vi "A170316-11_config.vi"() -> ()   [LabVIEW 2020]
uses:
  Global_Variable/Global.vi
  Database/Global1.vi
  <vilib>/Utility/config.llb/NI_LVConfig.lvlib
panel:
  in  "选项卡控件":enum32{"参数", "备用参数", "产品管理"}(tab)
  in  "参数设定":string[][](table)=[["", "", "", ""], ["", "", "", ""]]
  in  "删除":bool
  in  "确定":bool
  in  "添加":bool
  in  "退出":bool
  in  "更新":bool
  in  "产品型号":string(combo)
  in  "请输入添加的产品名称":string
  in  "请选择要删除的产品":string(combo)
  # "激光打标机"
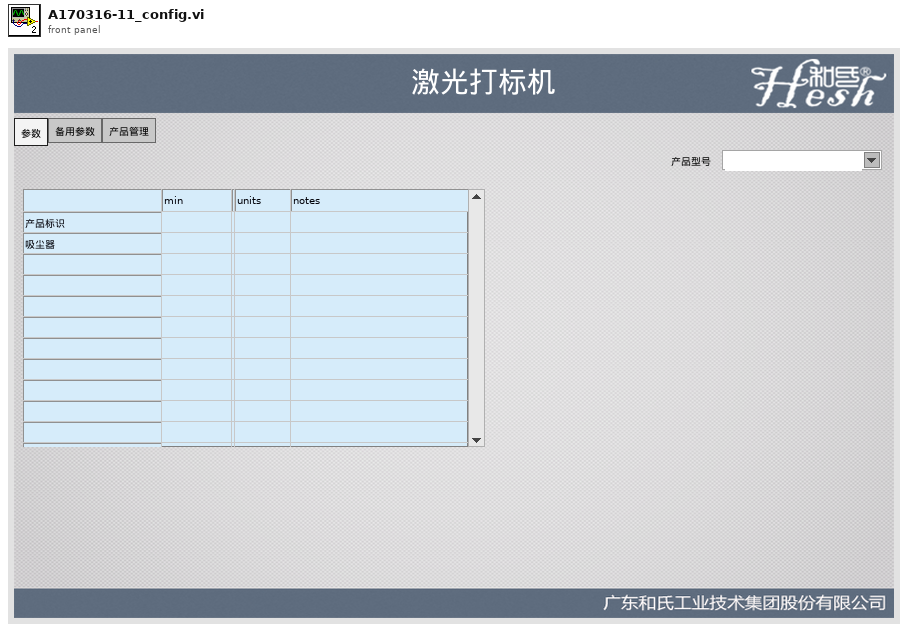
[diagram p1: front panel]
types:
  T1 = typedef "NI_LVConfig.lvlib/Config Data RefNum.ctl" = refnum<k1>
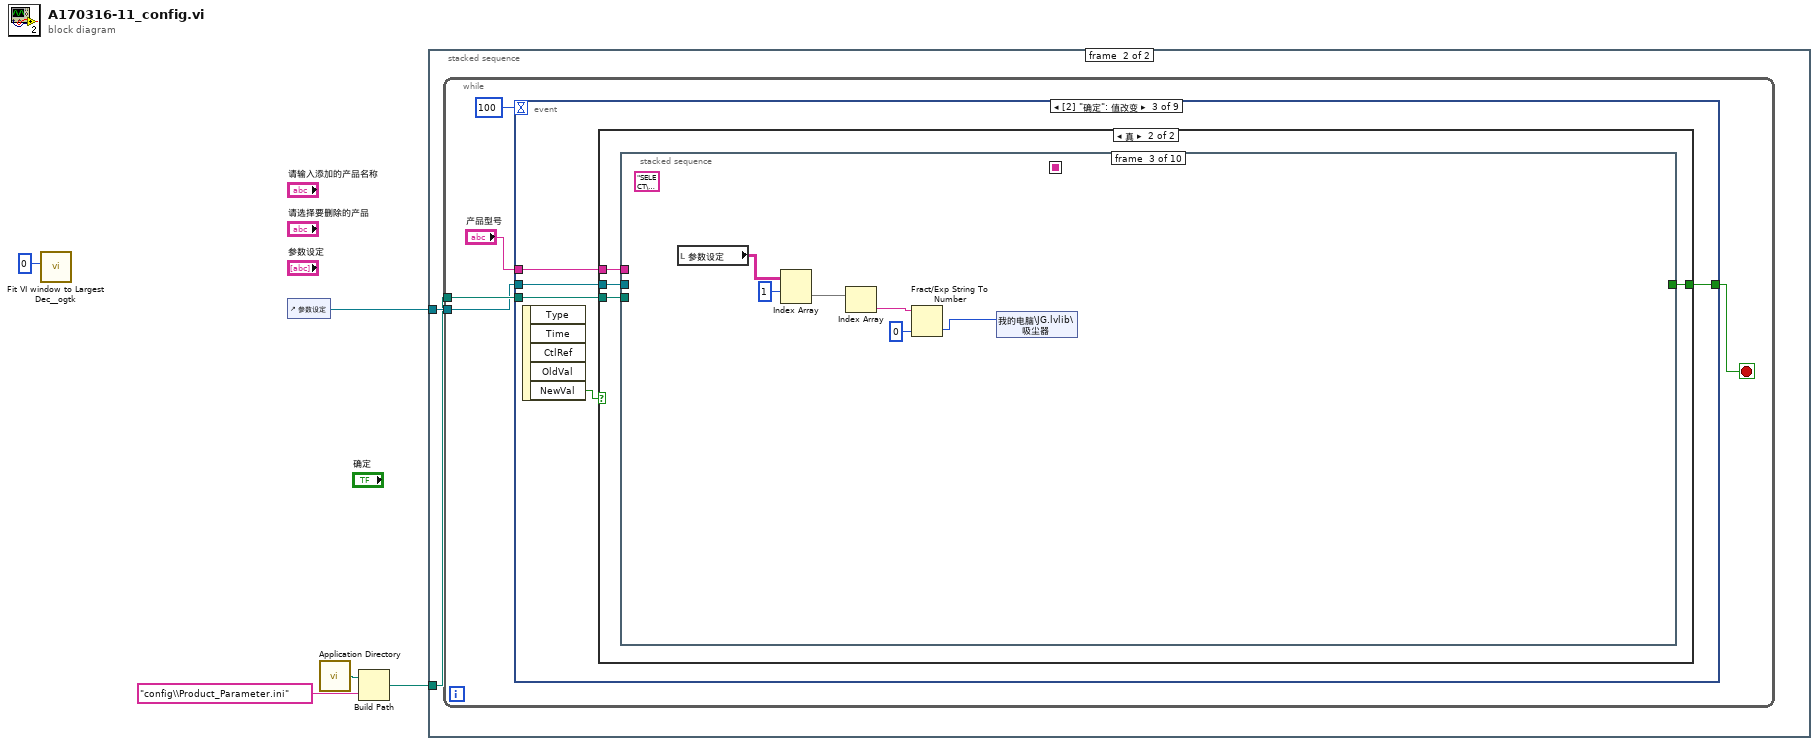
[diagram p0: block diagram]
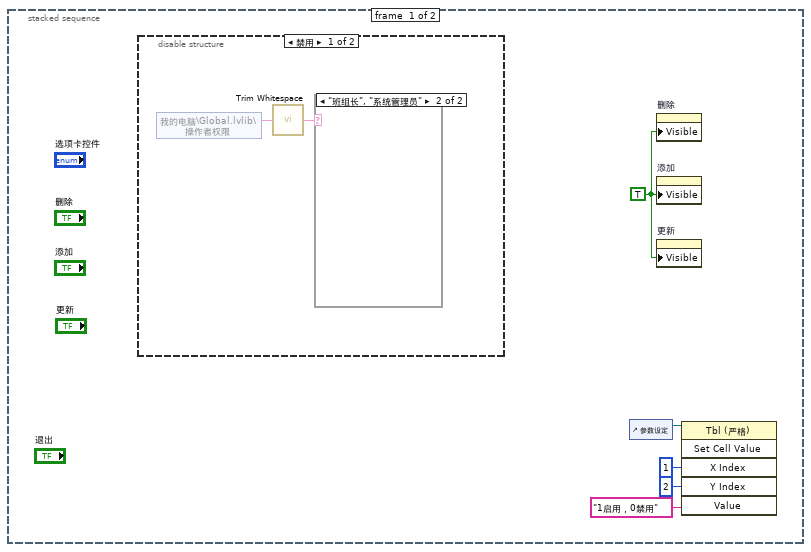
[diagram p2: hidden frame]
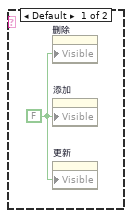
[diagram p3: hidden frame]
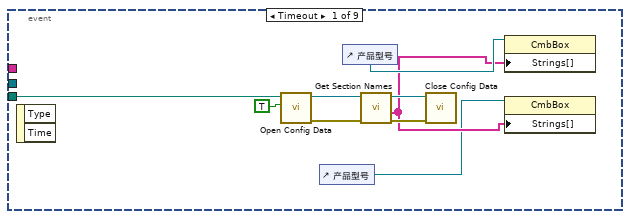
[diagram p5: hidden frame]
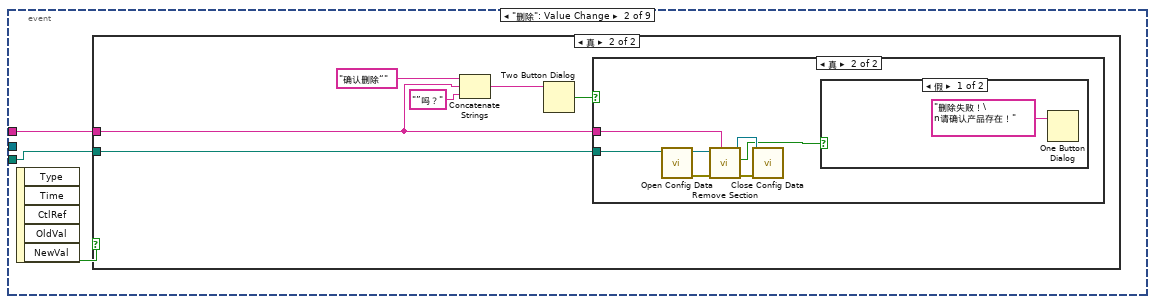
[diagram p6: hidden frame]
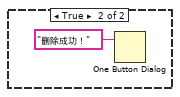
[diagram p9: hidden frame]
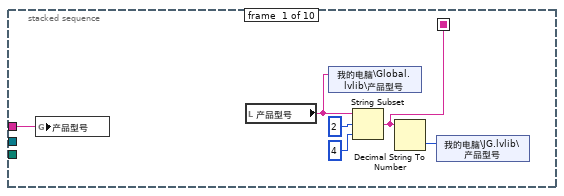
[diagram p11: hidden frame]
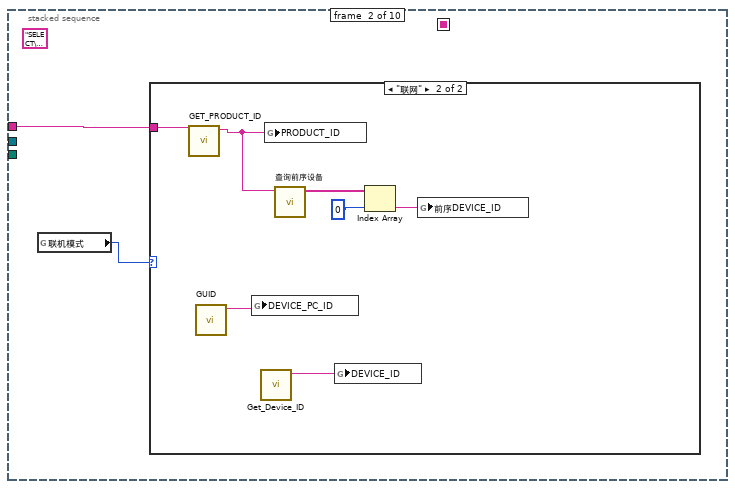
[diagram p12: hidden frame]
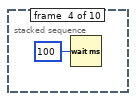
[diagram p14: hidden frame]
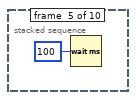
[diagram p15: hidden frame]
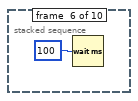
[diagram p16: hidden frame]
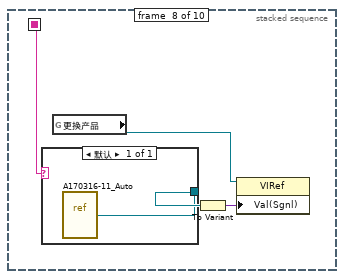
[diagram p18: hidden frame]
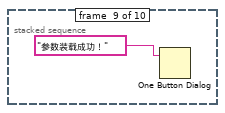
[diagram p19: hidden frame]
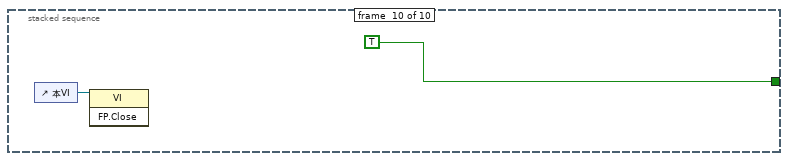
[diagram p20: hidden frame]
diagram:
  n1 = call <userlib>:"Fit VI window to Largest Dec__ogtk.vi"("border spacing (2 px)"=0) -> ()  [unwired: 5 in, 2 out]
  n2 = control-ref of="参数设定"() -> (w1:refnum<vi>)
  n3 = call <vilib>:"Application Directory.vi"() -> ("Application Directory"=w5:path)
  n4 = Build Path(base path=w5, name or relative path="config\\Product_Parameter.ini" ("名称或相对路径")) -> (appended path=w3:path)
  n5 = stacked-sequence {
    tunnel: w1 -> [_ w15]
    tunnel: w3 -> [_ w14]
    frame #0 {
      w10 = TRUE ("可见")
      n6 = disable-structure shown="禁用" {
        frame Disabled {
          n7 = shared-variable "我的电脑\\Global.lvlib\\操作者权限"() -> (w12:string)  [unwired: 1 in, 1 out]
          n8 = call <vilib>:"Trim Whitespace.vi"("string"=w12) -> ("trimmed string"=w11:string)  [unwired: 1 in]
          n9 = case shown="\"班组长\", \"系统管理员\"" w11 {
            frame Default {
              w13 = FALSE ("可见")
              n10 = property on="删除" class="Bool (严格)"("Visible"=w13) -> ()  [unwired: 2 in, 2 out]
              n11 = property on="添加" class="Bool (严格)"("Visible"=w13) -> ()  [unwired: 2 in, 2 out]
              n12 = property on="更新" class="Bool (严格)"("Visible"=w13) -> ()  [unwired: 2 in, 2 out]
            }
            frame "班组长", "系统管理员" {
            }
          }
        }
        frame Enabled {
        }
      }
      n13 = control-ref of="参数设定"() -> (w9:refnum<vi>)
      n14 = property on="删除" class="Bool (严格)"("Visible"=w10) -> ()  [unwired: 2 in, 2 out]
      n15 = property on="添加" class="Bool (严格)"("Visible"=w10) -> ()  [unwired: 2 in, 2 out]
      n16 = property on="更新" class="Bool (严格)"("Visible"=w10) -> ()  [unwired: 2 in, 2 out]
      n17 = invoke class="Tbl (严格)" method="Set Cell Value"(reference=w9, "X Index"=1 ("X索引"), "Y Index"=2 ("Y索引"), "Value"="1启用，0禁用" ("值")) -> ()  [unwired: 2 in, 6 out]
    }
    frame #1 {
      n18 = while {
        tunnel: w14 -> [w20]
        tunnel: w15 -> [w18]
        stop <- w19 stop-if-true
        n19 = event shown="[2] \"确定\": 值改变" {
          selector: _ -> [_ _ _ _ _ _ _ _ _]
          dyn-events: _ -> [_ _ _ _ _ _ _ _ _]
          timeout: 100 -> [_ _ _ _ _ _ _ _ _]
          tunnel: w20 -> [w24 w32 w49 w94 w110 _ w127 _ _]
          tunnel: [_ _ w51 _ _ TRUE _ _ TRUE] -> w19
          tunnel: w18 -> [_ _ w50 w95 w111 _ w126 _ _]
          tunnel: "产品型号" -> [_ w30 w48 w89 _ _ _ _ _]
          event Timeout {
            n20 = event-data() -> ()  [unwired: 1 in, 2 out]
            n21 = call <vilib>:"Open Config Data.vi"("create file if necessary (T)"=TRUE, "configuration file path"=w24) -> ("error out"=w26:errorcluster, "refnum"=w25:T1)  [unwired: 7 in, 1 out]
            n22 = control-ref of="产品型号"() -> (w21:refnum<vi>)
            n23 = control-ref of="产品型号"() -> (w23:refnum<vi>)
            n24 = call <vilib>:"Get Section Names.vi"("error in (no error)"=w26, "refnum"=w25) -> ("error out"=w28:errorcluster, "section names"=w22:string[], "refnum out"=w27:T1)  [unwired: 7 in]
            n25 = call <vilib>:"Close Config Data.vi"("error in (no error)"=w28, "refnum"=w27) -> ()  [unwired: 8 in, 2 out]
            n26 = property on="属性节点" class="CmbBox"(reference=w23, "Strings[]"=w22) -> ()  [unwired: 1 in, 2 out]
            n27 = property on="属性节点" class="CmbBox"(reference=w21, "Strings[]"=w22) -> ()  [unwired: 1 in, 2 out]
          }
          event "删除": Value Change {
            n28 = event-data() -> ("NewVal"=w31:bool)  [unwired: 1 in, 4 out]
            n29 = case shown="真" w31 {
              tunnel: w32 -> [_ w34]
              tunnel: w30 -> [_ w33]
              frame False {
              }
              frame True {
                n30 = Concatenate Strings("确认删除“", w33, "”吗？") -> (w36:string)
                n31 = Two Button Dialog(message=w36) -> (T button?=w35:bool)  [unwired: 2 in]
                n32 = case shown="真" w35 {
                  tunnel: w34 -> [_ w40]
                  tunnel: w33 -> [_ w39]
                  frame False {
                  }
                  frame True {
                    n33 = call <vilib>:"Open Config Data.vi"("configuration file path"=w40) -> ("error out"=w42:errorcluster, "refnum"=w45:T1)  [unwired: 8 in, 1 out]
                    n34 = call <vilib>:"Remove Section.vi"("section"=w39, "error in (no error)"=w42, "refnum"=w45) -> ("error out"=w44:errorcluster, "section exists?"=w41:bool, "refnum out"=w43:T1)  [unwired: 6 in]
                    n35 = call <vilib>:"Close Config Data.vi"("error in (no error)"=w44, "refnum"=w43) -> ()  [unwired: 8 in, 2 out]
                    n36 = case shown="假" w41 {
                      frame False {
                        n37 = One Button Dialog(message="删除失败！\n请确认产品存在！" ("消息")) -> ()  [unwired: 1 in, 1 out]
                      }
                      frame True {
                        n38 = One Button Dialog(message="删除成功！" ("消息")) -> ()  [unwired: 1 in, 1 out]
                      }
                    }
                  }
                }
              }
            }
          }
          event "确定": Value Change {
            n39 = event-data() -> ("NewVal"=w52:bool)  [unwired: 1 in, 4 out]
            n40 = case shown="真" w52 {
              tunnel: [_ w56] -> w51
              tunnel: w50 -> [_ w55]
              tunnel: w49 -> [_ w54]
              tunnel: w48 -> [_ w53]
              frame False {
              }
              frame True {
                n41 = stacked-sequence {
                  seq-local: [w62 _ _ _ _ _ _ _ _ _] -> [_ _ _ _ _ _ _ w84 _ _]
                  tunnel: [_ _ _ _ _ _ _ _ _ TRUE] -> w56
                  tunnel: w55 -> [_ _ _ _ _ _ _ _ _ _]
                  tunnel: w54 -> [_ _ _ _ _ _ _ _ _ _]
                  tunnel: w53 -> [w57 w64 _ _ _ _ _ _ _ _]
                  frame #0 {
                    n42 = global write "Global.vi" "产品型号"(w57) -> ()
                    n43 = local read "产品型号"() -> (w61:string)
                    n44 = shared-variable "我的电脑\\Global.lvlib\\产品型号"(w61) -> ()  [unwired: 1 in, 1 out]
                    n45 = String Subset(string=w61, offset (0)=u16 2 ("偏移量(0)"), length (rest)=u16 4 ("长度（剩余）")) -> (substring=w62:string)
                    n46 = Decimal String To Number(string=w62) -> (number=w58:i32)  [unwired: 2 in, 1 out]
                    n47 = shared-variable "我的电脑\\JG.lvlib\\产品型号"(w58) -> ()  [unwired: 1 in, 1 out]
                  }
                  frame #1 {
                    (unwired) "SELECT\ndbo.[Product].USER_ID\nFROM\ndbo.[Product]\nWHERE\ndbo.[Product].PRODUCT_NAME = '%s'" ("格式字符串")
                    n48 = global read "Global1.vi" "联机模式"() -> (w63:enum16{"单机", "联网"})
                    n49 = case shown="\"联网\"" w63 {
                      tunnel: w64 -> [_ w70]
                      frame "单机", Default {
                      }
                      frame "联网" {
                        n50 = call "GET_PRODUCT_ID.vi"("PRODFUCT_NAME"=w70) -> ("PRODUCT_ID"=w69:string)  [unwired: 10 in]
                        n51 = call "GUID.vi"() -> ("trimmed string"=w71:string)  [unwired: 11 in]
                        n52 = global write "Global1.vi" "DEVICE_PC_ID"(w71) -> ()
                        n53 = call "Get_Device_ID.vi"() -> ("Device_ID"=w65:string)  [unwired: 10 in, 1 out]
                        n54 = global write "Global1.vi" "PRODUCT_ID"(w69) -> ()
                        n55 = call "查询前序设备.vi"("PRODUCT_ID"=w69) -> ("前序工位"=w68:string[])  [unwired: 10 in]
                        n56 = global write "Global1.vi" "DEVICE_ID"(w65) -> ()
                        n57 = Index Array(array=w68, index=0 ("索引")) -> (element=w66:string)
                        n58 = global write "Global1.vi" "前序DEVICE_ID"(w66) -> ()
                      }
                    }
                  }
                  frame #2 {
                    (unwired) "SELECT\ndbo.[Product].USER_ID\nFROM\ndbo.[Product]\nWHERE\ndbo.[Product].PRODUCT_NAME = '%s'" ("格式字符串")
                    n59 = local read "参数设定"() -> (w77:string[][])
                    n60 = Index Array(array=w77, index (row)=1 ("索引 (行)")) -> (element=w76:string[])  [unwired: 1 in]
                    n61 = Index Array(array=w76) -> (element=w74:string)  [unwired: 1 in]
                    n62 = Fract/Exp String To Number(string=w74, default (0 dbl)=0 ("默认(0 DBL)")) -> (number=w73:i32)  [unwired: 2 in, 1 out]
                    n63 = shared-variable "我的电脑\\JG.lvlib\\吸尘器"(w73) -> ()  [unwired: 1 in, 1 out]
                  }
                  frame #3 {
                    n64 = Wait (ms)(milliseconds to wait=u32 100) -> ()  [unwired: 1 out]
                  }
                  frame #4 {
                    n65 = Wait (ms)(milliseconds to wait=u32 100) -> ()  [unwired: 1 out]
                  }
                  frame #5 {
                    n66 = Wait (ms)(milliseconds to wait=u32 100) -> ()  [unwired: 1 out]
                  }
                  frame #6 {
                  }
                  frame #7 {
                    n67 = case shown="默认" w84 {
                      tunnel: [w85] -> w81
                      frame 默认 {
                        n68 = vi-ref "A170316-11_Auto.vi"() -> (w85:refnum<vi>)
                      }
                    }
                    n69 = global read "Global.vi" "更换产品"() -> (w83:refnum<vi>)
                    n70 = To Variant(anything=w81) -> (Variant=w82:variant)
                    n71 = property class="VIRef"(reference=w83, "Val(Sgnl)"=w82) -> ()  [unwired: 1 in, 2 out]
                  }
                  frame #8 {
                    n72 = One Button Dialog(message="参数装载成功！" ("消息")) -> ()  [unwired: 1 in, 1 out]
                  }
                  frame #9 {
                    n73 = control-ref of="本VI"() -> (w87:refnum<vi>)
                    n74 = invoke class="VI" method="FP.Close"(reference=w87) -> ()  [unwired: 2 in, 3 out]
                  }
                }
              }
            }
          }
          event "添加": Value Change {
            n75 = event-data() -> ("NewVal"=w93:bool)  [unwired: 1 in, 4 out]
            n76 = local read "产品型号"() -> (w90:string)
            n77 = call <vilib>:"Trim Whitespace.vi"("string"=w90) -> ("trimmed string"=w91:string)  [unwired: 1 in]
            n78 = White Space?(1:w91) -> (0:w92:bool)
            n79 = case shown="假" w92 {
              tunnel: w95 -> [w99 _]
              tunnel: w94 -> [w98 _]
              tunnel: w93 -> [w97 _]
              tunnel: w89 -> [w96 _]
              frame False {
                n80 = case shown="假" w97 {
                  tunnel: w99 -> [_ w103]
                  tunnel: w98 -> [_ w102]
                  tunnel: w96 -> [_ w100]
                  frame False {
                  }
                  frame True {
                    n81 = call "Read_Write ParaINI File.vi"("Mode"=enum16{"Read", "Write"}."Write", "Section"=w100, "Filepath"=w102, "Ctl Refnum"=w103) -> ()  [unwired: 7 in, 1 out]
                  }
                }
              }
              frame True {
                w104 = 64 items=["None"=0, "Hand, Error, Stop"=16, "Question"=32, "Exclamation, Warning"=48, "Asterisk, Information"=64] ("icon")
                w105 = 0 items=["OK", "OKCancel", "AbortRetryIgnore", "YesNoCancel", "YesNo", "RetryCancel"] ("buttons")
                n82 = call "信息框（标题、文本、图标）.vi"("icon"=w104, "buttons"=w105, "caption"="添加失败", "text"="请输入产品名称!") -> ()  [unwired: 6 in, 2 out]
              }
            }
          }
          event "产品型号": Value Change {
            n83 = event-data() -> ("CtlRef"=w109:refnum<vi>, "NewVal"=w108:string)  [unwired: 1 in, 3 out]
            n84 = stacked-sequence {
              tunnel: w111 -> [_ w120]
              tunnel: w110 -> [_ w119]
              tunnel: w109 -> [w113 _]
              tunnel: w108 -> [w112 _]
              frame #0 {
                n85 = stacked-sequence {
                  tunnel: w113 -> [_ w115]
                  tunnel: w112 -> [_ w116]
                  frame #0 {
                    n86 = control-ref of="This VI"() -> (w114:refnum<vi>)
                    n87 = invoke class="VI" method="Default Vals.Reinit All"(reference=w114) -> ()  [unwired: 2 in, 3 out]
                  }
                  frame #1 {
                    n88 = property class="CmbBox"(reference=w115, "Value"=w116) -> ()  [unwired: 1 in, 2 out]
                  }
                }
              }
              frame #1 {
                n89 = local read "产品型号"() -> (w117:string)
                n90 = call "Read_Write ParaINI File.vi"("Mode"=enum16{"Read", "Write"}."Read", "Section"=w117, "Filepath"=w119, "Ctl Refnum"=w120) -> ()  [unwired: 7 in, 1 out]
              }
            }
          }
          event "退出": Value Change {
            n91 = event-data() -> ()  [unwired: 1 in, 5 out]
            n92 = control-ref of="本VI"() -> (w123:refnum<vi>)
            n93 = invoke class="VI" method="FP.Close"(reference=w123) -> (reference out=w121:refnum<vi>, error out=w122:errorcluster)  [unwired: 2 in, 1 out]
            n94 = Close Reference(reference=w121, error in (no error)=w122) -> ()  [unwired: 1 out]
          }
          event "更新": Value Change {
            n95 = event-data() -> ("NewVal"=w125:bool)  [unwired: 1 in, 4 out]
            n96 = case shown="真" w125 {
              tunnel: w127 -> [_ w132]
              tunnel: w126 -> [_ w131]
              frame False {
              }
              frame True {
                n97 = local read "产品型号"() -> (w129:string)
                n98 = call "Read_Write ParaINI File.vi"("Mode"=enum16{"Read", "Write"}."Write", "Section"=w129, "Filepath"=w132, "Ctl Refnum"=w131) -> ("error out"=w130:errorcluster)  [unwired: 7 in]
                n99 = case shown="无错误" w130 {
                  frame No Error {
                    n100 = call "浮动通知.vi"("通知内容"="更新成功！") -> ()  [unwired: 11 in]
                  }
                  frame Error {
                    n101 = call "浮动通知.vi"("通知内容"="更新失败！") -> ()  [unwired: 11 in]
                  }
                }
              }
            }
          }
          event "请输入添加的产品名称": Value Change {
            n102 = event-data() -> ("OldVal"=w137:string)  [unwired: 1 in, 5 out]
            n103 = control-ref of="产品型号"() -> (w135:refnum<vi>)
            n104 = property on="属性节点" class="CmbBox"(reference=w135) -> ("Strings[]"=w136:string[])  [unwired: 1 in, 2 out]
            n105 = for {
              tunnel: w137 -> [w138]
              tunnel: w136 -> [w139] mode=indexing
              n106 = Equal?(x=w138, y=w139) -> (x = y?=w140:bool)
              n107 = case shown="真" w140 {
                tunnel: w138 -> [_ w141]
                frame False {
                }
                frame True {
                  n108 = stacked-sequence {
                    tunnel: w141 -> [w147 _]
                    frame #0 {
                      w142 = 64 items=["None"=0, "Hand, Error, Stop"=16, "Question"=32, "Exclamation, Warning"=48, "Asterisk, Information"=64] ("icon")
                      w143 = 0 items=["OK", "OKCancel", "AbortRetryIgnore", "YesNoCancel", "YesNo", "RetryCancel"] ("buttons")
                      n109 = Concatenate Strings("已经存在产品”" ("text"), w147, "“\n请勿重复添加！" ("字符串")) -> (w145:string)
                      n110 = call "信息框（标题、文本、图标）.vi"("icon"=w142, "buttons"=w143, "caption"="产品重复", "text"=w145) -> ()  [unwired: 6 in, 2 out]
                    }
                    frame #1 {
                      n111 = local write "请输入添加的产品名称"("" ("请输入添加的产品名称")) -> ()
                    }
                  }
                }
              }
            }
          }
          event Panel Close {
            n112 = event-data() -> ()  [unwired: 1 in, 3 out]
          }
        }
      }
    }
  }
